vi "XML Script - Multiframe Structure.vi"   [LabVIEW 2017]
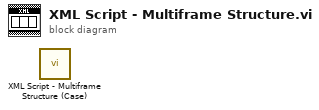
[diagram p0: block diagram]
diagram:
  n1 = call <vilib>:"XML Script - Multiframe Structure (Case).vi"() -> ()  [unwired: 10 in, 2 out]
